vi "Read Power.vi"(11 "RF Power in":refnum<class "RF Power.lvclass">) -> (2 "Power":cluster{"List":dbl[], "Index":i32, "Last":bool}, 3 "RF Power out":refnum<class "RF Power.lvclass">)   [LabVIEW 2020, in "RF Power.lvclass"]
uses:
  RF Power.lvclass
  RF Power.lvclass/RF Power.ctl
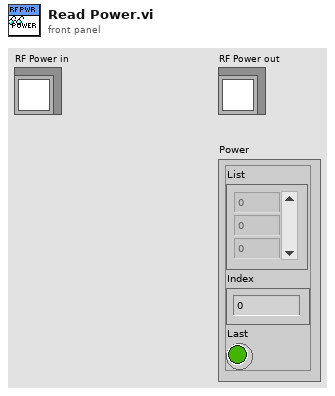
[diagram p1: front panel]
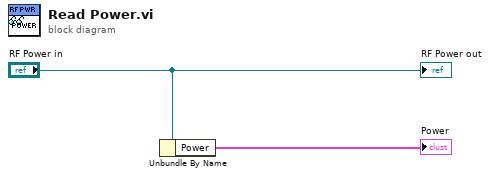
[diagram p0: block diagram]
diagram:
  n1 = Unbundle By Name("RF Power in") -> ("Power"=→"Power":cluster{"List":dbl[], "Index":i32, "Last":bool})
  "RF Power out" <- "RF Power in"
